vi "Format Value String.vi"(8 "error in (no error)":errorcluster, 11 "Data":variant) -> (0 "error out":errorcluster, 2 "Value as String":string)   [LabVIEW 2019, in "VariantExtensions.lvlib"]
doc: "<License>\nCopyright © 2017 Composed Systems, LLC | All rights reserved\nwww.composed.io\n\nAuthor: Ethan Stern <ethan.stern@composed.io>\n\nThis software is provided \"AS IS\" WITHOUT WARRANTIES, either express or implied, AND IS FOR EDUCATIONAL PURPOSES ONLY.\n</License>"
uses:
  <vilib>/gpm_packages/@cs/variant/Source/VariantExtensions.lvlib
  <vilib>/Utility/Data Type/Get Refnum Information.vi
  <vilib>/Utility/Data Type/NI_Data Type.lvlib
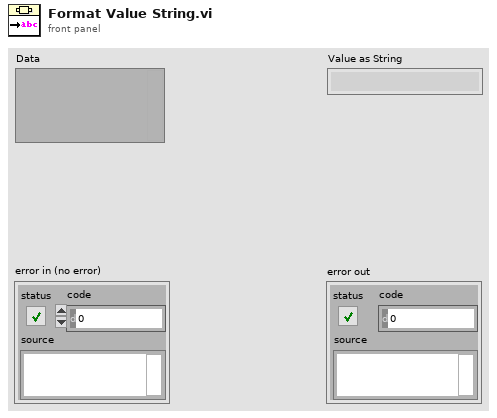
[diagram p1: front panel]
types:
  T1 = typedef "NI_Data Type.lvlib/Data Type.ctl" = enum8{"Invalid Type", "Void", "I8", "I16", "I32", "I64", "U8", "U16", "U32", "U64", "Single Float", "Double Float", "Extended Float", "Single Complex", "Double Complex", "Extended Complex", "Enum U8", "Enum U16", "Enum U32", "Enum U64", "Single Float With Unit", "Double Float With Unit", "Extended Float With Unit", "Single Complex with Unit", "Double Complex with Unit", "Extended Complex with Unit", "Boolean", "String", "Path", "Picture", "Tag", "Array", "Cluster", "Variant", "LV Variant", "Waveform", "Timestamp", "Digital Waveform", "Digital Data", "ExpressData", "Refnum", "External Data", "VI", "Poly VI", "LabVIEW Class Instance", "Fixed Point", "Set Collection", "Map Collection"}
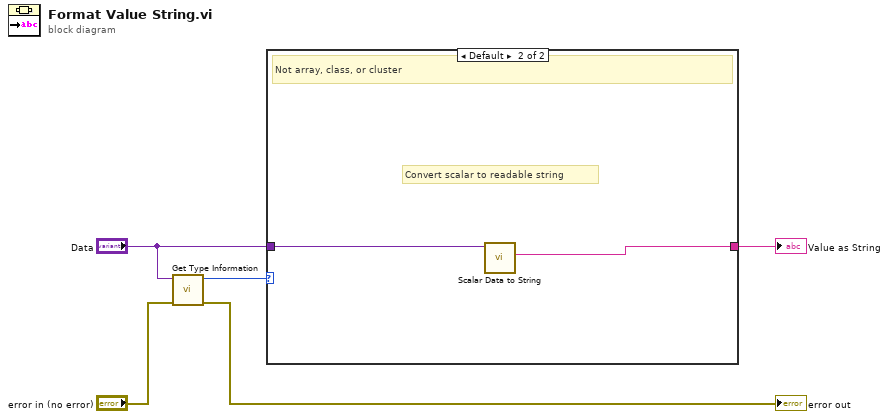
[diagram p0: block diagram]
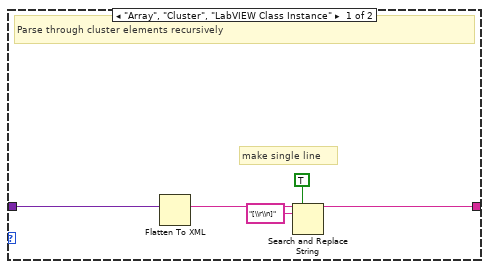
[diagram p2: hidden frame]
diagram:
  n1 = call <vilib>:"Get Type Information.vi"("error in (no error)"="error in (no error)", "variant"="Data") -> ("error out"=→"error out":errorcluster, "type"=w4:T1)  [unwired: 5 in, 3 out]
  n2 = case shown="Default" w4 {
    tunnel: [w10 w12] -> w5
    tunnel: "Data" -> [w9 w11]
    frame "Array", "Cluster", "LabVIEW Class Instance" {
      # "make single line"
      # "Parse through cluster elements recursively"
      n3 = Flatten To XML(anything=w9) -> (xml string=w8:string)
      n4 = Search and Replace String(replace all?=TRUE ("replace all? (F)"), input string=w8, search string="[\\r\\n]") -> (result string=w10:string)  [unwired: 5 in, 3 out]
    }
    frame Default {
      # "Convert scalar to readable string"
      # "Not array, class, or cluster"
      n5 = call <vilib>:"Scalar Data to String.vi"("Data"=w11) -> ("Value String"=w12:string)  [unwired: 9 in, 1 out]
    }
  }
  "Value as String" <- w5
